vi "Main.vi"(8 "error in":errorcluster, 10 "Sequence Context":refnum<k7>, 11 "OPC UA In":refnum<class "Abstract UUT.lvclass">) -> (0 "error out":errorcluster, 3 "OPC UA Out":refnum<class "Abstract UUT.lvclass">)   [LabVIEW 2019, in "Sequence Main.lvlib" / "Abstract UUT.lvclass"]
uses:
  Abstract UUT.lvclass
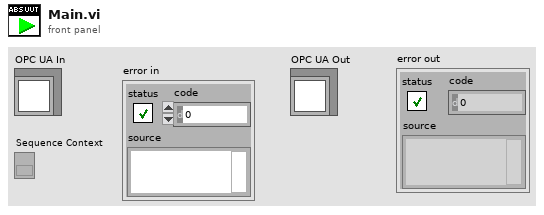
[diagram p1: front panel]
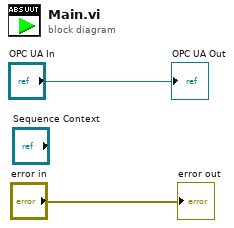
[diagram p0: block diagram]
diagram:
  "error out" <- "error in"
  "OPC UA Out" <- "OPC UA In"
